vi "Read Text File.vi"(8 "error in":errorcluster, 11 "File Path":path) -> (0 "error out":errorcluster, 3 "Data Out":dbl[][](array[numeric]) format="%0.2f")   [LabVIEW 2021]
doc: "Reads data from a .txt file."
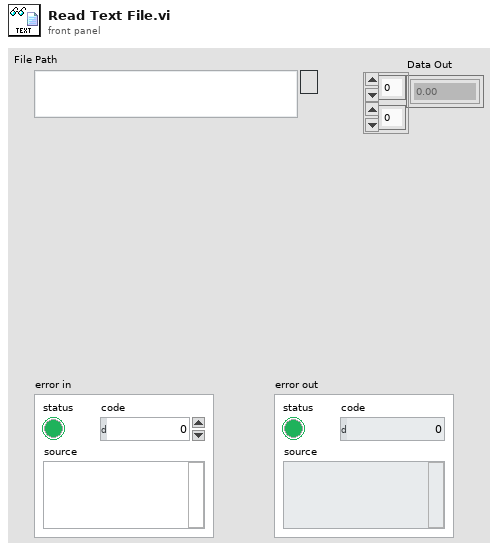
[diagram p1: front panel]
types:
  T1 = enum16{"open", "replace", "create", "open or create", "replace or create", "replace or create with confirmation"}
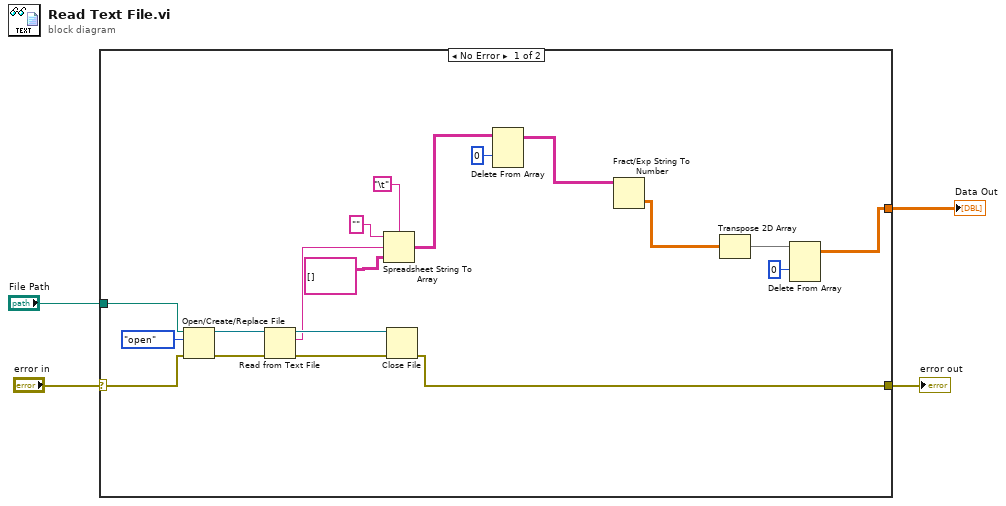
[diagram p0: block diagram]
diagram:
  n1 = case shown="No Error" "error in" {
    selector: "error in" -> [w21 w24]
    tunnel: [w16 w24] -> w3
    tunnel: "File Path" -> [w22 _]
    tunnel: [w7 _] -> w1
    frame No Error {
      n2 = Open/Create/Replace File(file path (use dialog)=w22, error in=w21, operation (0:open)=T1."open") -> (refnum out=w20:refnum<file>, error out=w19:errorcluster)  [unwired: 3 in, 1 out]
      n3 = Read from Text File(file (use dialog)=w20, error in=w19) -> (refnum out=w18:refnum<file>, text=w15:string, error out=w17:errorcluster)  [unwired: 2 in, 1 out]
      n4 = Spreadsheet String To Array(delimiter (Tab)="\t", format string="", spreadsheet string=w15, array type (2D Dbl)=string[][] []) -> (array=w11:string[][])
      n5 = Close File(refnum=w18, error in=w17) -> (error out=w16:errorcluster)  [unwired: 1 out]
      n6 = Delete From Array(array=w11, index (row)=0) -> (array with subset deleted=w5:string[][])  [unwired: 2 in, 1 out]
      n7 = Fract/Exp String To Number(string=w5) -> (number=w9:dbl[][])  [unwired: 3 in, 1 out]
      n8 = Transpose 2D Array(2D array=w9) -> (transposed array=w8:dbl[][])
      n9 = Delete From Array(array=w8, index (row)=0) -> (array with subset deleted=w7:dbl[][])  [unwired: 2 in, 1 out]
    }
    frame Error {
    }
  }
  "error out" <- w3
  "Data Out" <- w1
